vi "Remote Communication.vi"(4 "String":string, 5 "Max Mass":dbl, 6 "Error In":errorcluster, 7 "DC Param":u16, 8 "RT Parameter":T1 {"Expt"."Mass Range"."Resolution Type" items=["High/High", "Medium/Medium", "Low/Low", "High/Medium", "High/Low", "Medium/High", "Medium/Low", "Low/High", "Low/Medium"]}, 9 "Command":T7=enum."Start") -> (0 "Error Out":errorcluster, 1 "Data Array":i32[](array[numeric]), 2 "Info":string, 3 "Comm Error":bool)   [LabVIEW 2018]
doc: "This VI use TCP IP to communicate with RT"
uses:
  Type Defs/RT Command.ctl
  RT Parameters/RT Parameter.ctl
  RT Parameters/RT Experiments.ctl
  RT Parameters/RT Mass Range.ctl
  RT Parameters/RT Active Ch.ctl
  RT Parameters/RT Res Type.ctl
  RT Parameters/RT Run Mode.ctl
  Type Defs/Global Action.ctl
  Type Defs/TCP Packet Info.ctl
  Type Defs/RT Data.ctl
  FGVs/Global Variables.vi
panel:
  out "Number Matched":bool
  in  "IP Address":string
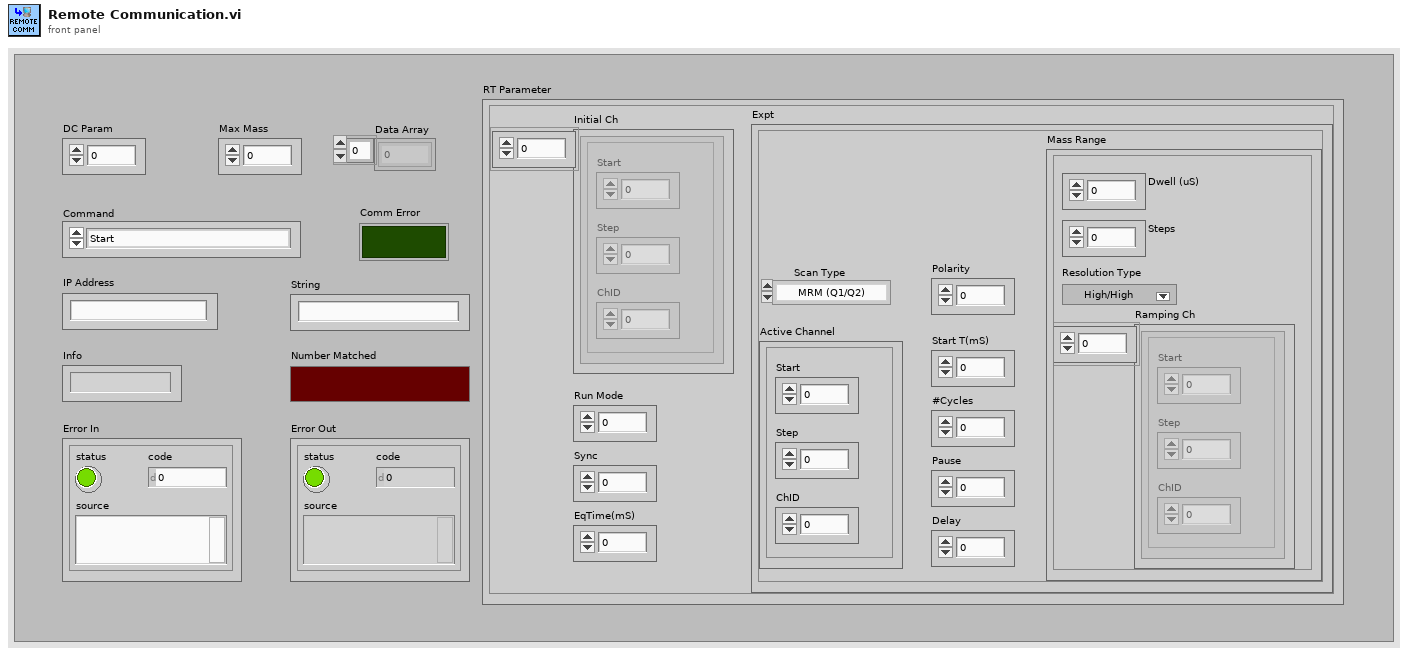
[diagram p1: front panel]
types:
  T1 = typedef "RT Parameter.ctl" = cluster{"Expt":T2, "Initial Ch":T4[], "Run Mode":i32, "Sync":u8, "EqTime(mS)":i32}
  T2 = typedef "RT Experiments.ctl" = cluster{"Mass Range":T3, "Active Channel":T4, "Scan Type":T6, "Polarity":u8, "Start T(mS)":i32, "#Cycles":i32, "Pause":i32, "Delay":i32}
  T3 = typedef "RT Mass Range.ctl" = cluster{"Ramping Ch":T4[], "Resolution Type":T5, "Steps":dbl, "Dwell (uS)":dbl}
  T4 = typedef "RT Active Ch.ctl" = cluster{"Start":dbl, "Step":dbl, "ChID":dbl}
  T5 = typedef "RT Res Type.ctl" = u16
  T6 = typedef "RT Run Mode.ctl" = enum16{"MRM (Q1/Q2)", "Q1 Scan", "Q1 SRM", "Q2 Scan", "Q2 SRM", "Product Scan", "Precursor Scan", "Neutral Loss", "Neutral Gain"}
  T7 = typedef "RT Command.ctl" = enum16{"xml Start Run", "xml Start Actual Run", "xml Stop Run", "xml Runtime Update", "xml Get Status", "xml Get Table", "xml Set Table", "xml Get Configuration", "xml System Status", "xml Set LC Input Logic", "xml Get Data", "xml Get Info", "Start", "StartActualRun", "Stop", "Runtime Update", "Get Data", "Get Info", "Get Status", "Get Param", "Get Config", "Get Table", "Read ADC", "Set Oscillator", "Update Config", "Update Table", "Set All Pol", "Set Pol and DC", "Set Max Mass", "Toggle RP", "Toggle EL", "Set PIC", "Initialize Turbo", "Send Turbo Comm", "Close Turbo", "P1", "P2", "P3", "Send Serial", "Set LC Out", "Get LC In", "Read VAC", "Test Table", "Toggle Power", "Get Startup", "Set Startup", "Get ADC Table", "Set ADC Table", "Get Brief Status", "Get Detail Status", "Auxiliary Update", "Set CC Logics", "Set CC Input Logics", "Ignore Error", "invalid"}
  T8 = typedef "TCP Packet Info.ctl" = cluster{"Packet Signature":string, "Sequence Number":i32, "Command":T7, "Data Message Size":u32, "Data Message Size":string, "Data Message":string, "Error Message Size":u32, "Error Message Size":string, "Error Message":string, "Checksum":u32, "Error Message":errorcluster, "Command ID":string}
  T9 = typedef "Global Action.ctl" = enum16{"Write", "Read"}
  T10 = typedef "RT Data.ctl" = cluster{"Info":string, "Data Array":i32[], "error out":errorcluster}
  T11 = typedef "Global Configrations.ctl" = cluster{"Model Name":enum16{"QSight 110", "QSight 120", "QSight 210", "QSight 220", "QSight 410", "QSight 420", "IONICS 3Q 110", "IONICS 3Q 120", "IONICS 3Q 210", "IONICS 3Q 220", "IONICS 3Q 310", "IONICS 3Q 320", "Simulation (Single Source)", "Simulation (Dual Source)"}, "RunType":u16, "Acquisition State":enum16{"Ready", "Busy", "Waiting"}, "InstrState":enum16{"Initializing", "Mass Spectrometer is Off", "Starting Up", "Turning Power Off", "Going to Standby", "Roughing Pump Ready", "Turning Turbo Off", "Turbo Startup", "Turbopump Ready", "Checking Vacuum", "Going to Ready", "Ready", "Running", "Source Standby", "Lost Communication", "Shutting Down", "Fault", "24V Standby", "Go to 24V Standby", "Turbopump Ready-Waiting"}, "Run Mode":enum16{"MRM (Q1/Q2)", "Q1 Scan", "Q1 SRM", "Q2 Scan", "Q2 SRM", "Product Scan", "Precursor Scan", "Neutral Loss", "Neutral Gain"}, "Configration":T12, "TCP ID":refnum<k5>, "DT":bool, "Dead Time (nS)":i32, "Single Source":bool, "ADC Tables":T14[]}
  T12 = typedef "Configration.ctl" = cluster{"Table":T13[], "Instrument":string[]}
  T13 = typedef "_RT Configuration 2.ctl" = cluster{"Name":string, "Ch#":u8, "Min":dbl, "Max":dbl, "Def+":dbl, "Def-":dbl, "Offset":dbl, "Slope":dbl, "Type":u8, "Description":string, "SettleT":dbl}
  T14 = typedef "ADC Table.ctl" = cluster{"Name":string, "Ch#":u8, "Min":dbl, "Max":dbl, "Def+":dbl, "Def-":dbl, "Offset":dbl, "Slope":dbl, "Type":u8, "Description":string, "SettleT":dbl}
  T15 = typedef "Global Parameters.ctl" = cluster{"Calibrations":cluster{"Q1 +ve":dbl[][], "Q2 +ve":dbl[][], "Q1 -ve":dbl[][], "Q2 -ve":dbl[][]}, "Resolution Q1":cluster{"High +ve":dbl[][], "Med +ve":dbl[][], "Low +ve":dbl[][], "High -ve":dbl[][], "Med -ve":dbl[][], "Low -ve":dbl[][]}, "Resolution Q2":cluster{"High +ve":dbl[][], "Med +ve":dbl[][], "Loe +ve":dbl[][], "High -ve":dbl[][], "Med -ve":dbl[][], "Low -ve":dbl[][]}, "MR Parameters":T16, "Mass":dbl[][], "Dwell":dbl[][], "Steps":i32[][], "Method Refnum":refnum<vi>}
  T16 = typedef "MR Parameters.ctl" = cluster{"Name":string, "Ch#":u8, "StartV":dbl, "StopV":dbl, "StepV":dbl, "Index":u8}
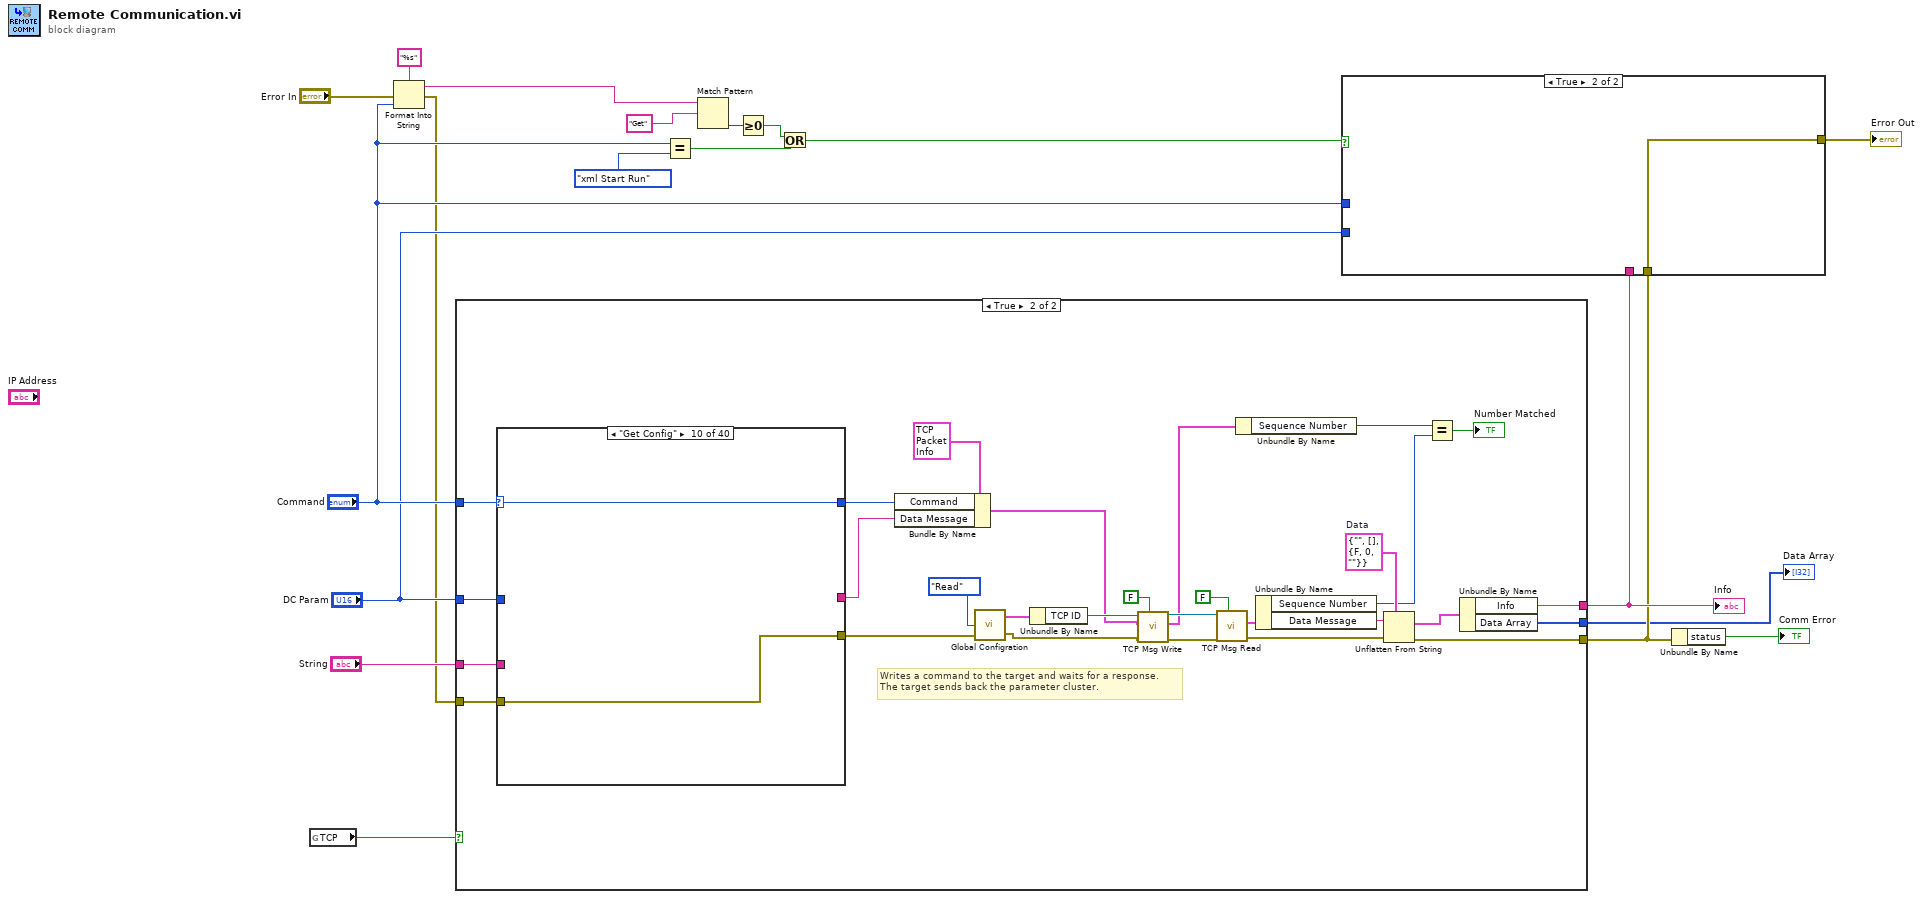
[diagram p0: block diagram]
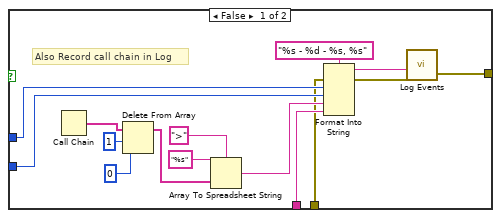
[diagram p2: hidden frame]
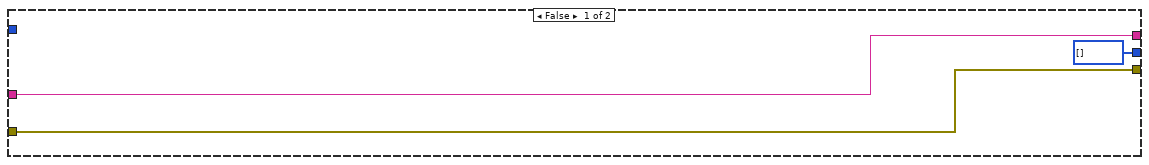
[diagram p3: hidden frame]
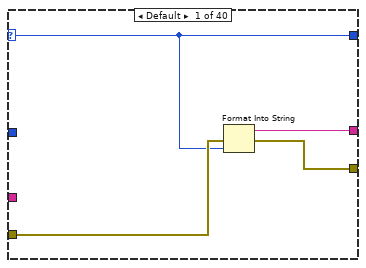
[diagram p4: hidden frame]
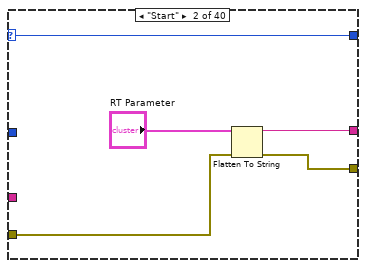
[diagram p5: hidden frame]
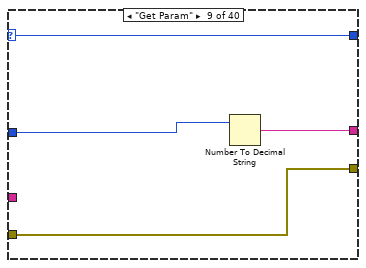
[diagram p12: hidden frame]
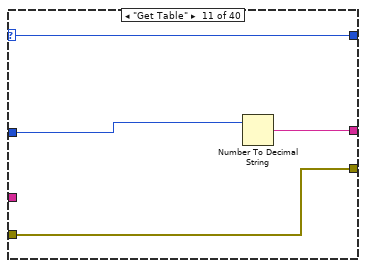
[diagram p13: hidden frame]
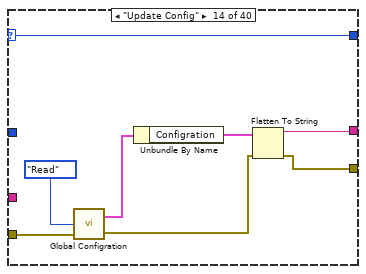
[diagram p16: hidden frame]
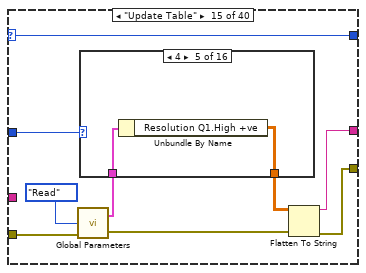
[diagram p17: hidden frame]
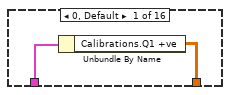
[diagram p18: hidden frame]
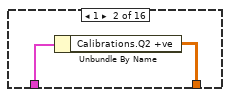
[diagram p19: hidden frame]
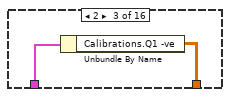
[diagram p20: hidden frame]
diagram:
  n1 = global read "Global Variables.vi" "TCP"() -> (w18:bool)
  n2 = Format Into String(format string="%s", error in="Error In", "Command") -> (resulting string=w6:string, error out=w5:errorcluster)  [unwired: 1 in]
  n3 = case shown="True" w18 {
    tunnel: "Command" -> [_ w51]
    tunnel: w5 -> [w22 w34]
    tunnel: "String" -> [w21 w48]
    tunnel: "DC Param" -> [_ w49]
    tunnel: [w22 w27] -> w3
    tunnel: [i32[] [] ("Data Array") w40] -> w1
    tunnel: [w21 w39] -> w8
    frame False {
    }
    frame True {
      w43 = T10 {"Info"="", "Data Array"=[], "error out"={"status"=FALSE, "code"=0, "source"=""}}  # Data
      # "Writes a command to the target and waits for a response.\nThe target sends back the parameter cluster."
      n4 = case shown="\"Get Config\"" w51 {
        selector: w51 -> [w53 w57 w62 w64 w65 w69 w71 w73 w77 w79 w80 w85 w88 w90 w98 w138 w143 w146 w153 w157 w160 w161 w165 w169 w174 w178 w180 w182 w183 w186 w191 w194 w196 w197 w200 w204 w205 w211 w215 w217]
        tunnel: [w53 w57 w62 w64 w65 w69 w71 w73 w77 w79 w80 w85 w88 w90 w98 w138 w143 w146 w153 w157 w160 w161 w165 w169 w174 w178 w180 w182 w183 w186 w191 w194 w196 w197 w200 w204 w205 w211 w215 w217] -> w50
        tunnel: w49 -> [_ _ _ _ _ _ _ _ w75 _ w82 _ _ _ w105 w140 w145 _ w150 w154 _ w163 w167 w171 _ w176 _ _ _ w188 _ _ _ _ _ _ _ w209 w213 w218]
        tunnel: w48 -> [_ _ _ _ w67 _ _ _ _ _ _ _ w87 _ _ _ _ _ _ _ w158 _ _ _ _ _ _ _ w185 _ _ w193 _ w199 w202 _ w206 _ _ _]
        tunnel: [w55 w60 _ _ w67 _ _ _ w76 _ w83 _ w87 w92 w100 w141 w144 w149 w151 w155 w158 w164 w168 w172 _ w177 _ _ w185 w189 _ w193 _ w199 w202 _ w206 w210 w214 w219] -> w47
        tunnel: w34 -> [w54 w58 w61 w63 w66 w68 w70 w72 w74 w78 w81 w84 w86 w93 w103 w139 w142 w147 w152 w156 w159 w162 w166 w170 w173 w175 w179 w181 w184 w187 w190 w192 w195 w198 w201 w203 w207 w208 w212 w216]
        tunnel: [w52 w59 w61 w63 w66 w68 w70 w72 w74 w78 w81 w84 w86 w91 w101 w139 w142 w147 w152 w156 w159 w162 w166 w170 w173 w175 w179 w181 w184 w187 w190 w192 w195 w198 w201 w203 w207 w208 w212 w216] -> w33
        frame Default {
          n5 = Format Into String(error in=w54, w53) -> (resulting string=w55:string, error out=w52:errorcluster)  [unwired: 2 in]
        }
        frame "Start" {
          n6 = Flatten To String(anything="RT Parameter", error in (no error)=w58) -> (data string=w60:string, error out=w59:errorcluster)  [unwired: 3 out]
        }
        frame "StartActualRun" {
        }
        frame "Stop" {
        }
        frame "Runtime Update" {
        }
        frame "Get Data" {
        }
        frame "Get Info" {
        }
        frame "Get Status" {
        }
        frame "Get Param" {
          n7 = Number To Decimal String(number=w75) -> (decimal integer string=w76:string)  [unwired: 1 out]
        }
        frame "Get Config" {
        }
        frame "Get Table" {
          n8 = Number To Decimal String(number=w82) -> (decimal integer string=w83:string)  [unwired: 1 out]
        }
        frame "Read ADC" {
        }
        frame "Set Oscillator" {
        }
        frame "Update Config" {
          n9 = call "Global Configration.vi"("Error In"=w93, "Action"=Global_Action."Read") -> ("Error Out"=w95:errorcluster, "Parameters Out"=w96:T11)  [unwired: 1 in]
          n10 = Unbundle By Name(w96) -> ("Configration"=w94:T12)
          n11 = Flatten To String(anything=w94, error in (no error)=w95) -> (data string=w92:string, error out=w91:errorcluster)  [unwired: 3 out]
        }
        frame "Update Table" {
          n12 = call "Global Parameters.vi"("Error In"=w103, "Action"=Global_Action."Read") -> ("Error Out"=w102:errorcluster, "Parameters Out"=w104:T15)  [unwired: 1 in]
          n13 = case shown="4" w105 {
            tunnel: w104 -> [w107 w109 w111 w112 w114 w116 w118 w120 w122 w124 w126 w128 w130 w132 w134 w136]
            tunnel: [w106 w108 w110 w113 w115 w117 w119 w121 w123 w125 w127 w129 w131 w133 w135 w137] -> w99
            frame 0, Default {
              n14 = Unbundle By Name(w107) -> ("Calibrations.Q1 +ve"=w106:dbl[][])
            }
            frame 1 {
              n15 = Unbundle By Name(w109) -> ("Calibrations.Q2 +ve"=w108:dbl[][])
            }
            frame 2 {
              n16 = Unbundle By Name(w111) -> ("Calibrations.Q1 -ve"=w110:dbl[][])
            }
            frame 3 {
              n17 = Unbundle By Name(w112) -> ("Calibrations.Q2 -ve"=w113:dbl[][])
            }
            frame 4 {
              n18 = Unbundle By Name(w114) -> ("Resolution Q1.High +ve"=w115:dbl[][])
            }
            frame 5 {
              n19 = Unbundle By Name(w116) -> ("Calibrations.Q1 +ve"=w117:dbl[][])
            }
            frame 6 {
              n20 = Unbundle By Name(w118) -> ("Calibrations.Q1 +ve"=w119:dbl[][])
            }
            frame 7 {
              n21 = Unbundle By Name(w120) -> ("Calibrations.Q1 +ve"=w121:dbl[][])
            }
            frame 8 {
              n22 = Unbundle By Name(w122) -> ("Calibrations.Q1 +ve"=w123:dbl[][])
            }
            frame 9 {
              n23 = Unbundle By Name(w124) -> ("Calibrations.Q1 +ve"=w125:dbl[][])
            }
            frame 10 {
              n24 = Unbundle By Name(w126) -> ("Calibrations.Q1 +ve"=w127:dbl[][])
            }
            frame 11 {
              n25 = Unbundle By Name(w128) -> ("Calibrations.Q1 +ve"=w129:dbl[][])
            }
            frame 12 {
              n26 = Unbundle By Name(w130) -> ("Calibrations.Q1 +ve"=w131:dbl[][])
            }
            frame 13 {
              n27 = Unbundle By Name(w132) -> ("Calibrations.Q1 +ve"=w133:dbl[][])
            }
            frame 14 {
              n28 = Unbundle By Name(w134) -> ("Calibrations.Q1 +ve"=w135:dbl[][])
            }
            frame 15 {
              n29 = Unbundle By Name(w136) -> ("Calibrations.Q1 +ve"=w137:dbl[][])
            }
          }
          n30 = Flatten To String(anything=w99, error in (no error)=w102) -> (data string=w100:string, error out=w101:errorcluster)  [unwired: 3 out]
        }
        frame "Set All Pol" {
          n31 = Type Cast(x=w140) -> (*(type *) &x=w141:string)  [unwired: 1 in]
        }
        frame "Set Pol and DC" {
          n32 = Type Cast(x=w145) -> (*(type *) &x=w144:string)  [unwired: 1 out]
        }
        frame "Set Max Mass" {
          n33 = Type Cast(x="Max Mass") -> (*(type *) &x=w149:string)  [unwired: 1 in]
        }
        frame "Toggle RP" {
          n34 = Number To Decimal String(number=w150) -> (decimal integer string=w151:string)  [unwired: 1 out]
        }
        frame "Toggle EL" {
          n35 = Number To Decimal String(number=w154) -> (decimal integer string=w155:string)  [unwired: 1 out]
        }
        frame "Set PIC" {
        }
        frame "P1" {
          n36 = Type Cast(x=w163) -> (*(type *) &x=w164:string)  [unwired: 1 in]
        }
        frame "P2" {
          n37 = Type Cast(x=w167) -> (*(type *) &x=w168:string)  [unwired: 1 in]
        }
        frame "P3" {
          n38 = Type Cast(x=w171) -> (*(type *) &x=w172:string)  [unwired: 1 in]
        }
        frame "Send Serial" {
        }
        frame "Set LC Out" {
          n39 = Type Cast(x=w176) -> (*(type *) &x=w177:string)  [unwired: 1 in]
        }
        frame "Get LC In" {
        }
        frame "Read VAC" {
        }
        frame "Test Table" {
        }
        frame "Toggle Power" {
          n40 = Number To Decimal String(number=w188) -> (decimal integer string=w189:string)  [unwired: 1 out]
        }
        frame "Get Startup" {
        }
        frame "Set Startup" {
        }
        frame "Get ADC Table" {
        }
        frame "Set ADC Table" {
        }
        frame "Get Brief Status" {
        }
        frame "Get Detail Status" {
        }
        frame "Auxiliary Update" {
        }
        frame "Set CC Logics" {
          n41 = Type Cast(x=w209) -> (*(type *) &x=w210:string)  [unwired: 1 in]
        }
        frame "Set CC Input Logics" {
          n42 = Type Cast(x=w213) -> (*(type *) &x=w214:string)  [unwired: 1 in]
        }
        frame "Ignore Error" {
          n43 = Number To Decimal String(number=w218) -> (decimal integer string=w219:string)  [unwired: 1 out]
        }
      }
      n44 = Bundle By Name(cluster=T8 {"Packet Signature"="", "Sequence Number"=0, "Command"=enum."Get Info", "Data Message Size"=0, "Data Message Size"="", "Data Message"="", "Error Message Size"=0, "Error Message Size"="", "Error Message"="", "Checksum"=0, "Error Message"={"status"=FALSE, "code"=0, "source"=""}, "Command ID"=""} ("Packet Info In Out 2"), "Command"=w50, "Data Message"=w47) -> (w36:T8)
      n45 = call "Global Configration.vi"("Error In"=w33, "Action"=Global_Action."Read") -> ("Error Out"=w38:errorcluster, "Parameters Out"=w46:T11)  [unwired: 1 in]
      n46 = Unbundle By Name(w46) -> ("TCP ID"=w37:refnum<k5>)
      n47 = call "TCP Msg Write.vi"("RT"=FALSE, "error in"=w38, "Packet Info In"=w36, "connection ID In"=w37) -> ("error out"=w32:errorcluster, "Packet Info In Out"=w24:T8, "connection ID out"=w28:refnum<k5>)  [unwired: 5 in]
      n48 = call "TCP Msg Read.vi"("RT"=FALSE, "error in"=w32, "connection ID"=w28) -> ("error out"=w30:errorcluster, "Packet Info"=w31:T8)  [unwired: 5 in, 2 out]
      n49 = Unbundle By Name(w24) -> ("Sequence Number"=w25:i32)
      n50 = Unbundle By Name(w31) -> ("Sequence Number"=w23:i32, "Data Message"=w42:string)
      n51 = Unflatten From String(type=w43, binary string=w42, error in (no error)=w30) -> (value=w41:T10, error out=w27:errorcluster)  [unwired: 3 out]
      n52 = Equal?(x=w25, y=w23) -> (x = y?=→"Number Matched":bool)
      n53 = Unbundle By Name(w41) -> ("Info"=w39:string, "Data Array"=w40:i32[])
    }
  }
  "Info" <- w8
  "Data Array" <- w1
  n54 = Equal?(x="Command", y=RT_Command."xml Start Run" ("RT Command")) -> (x = y?=w13:bool)
  n55 = Match Pattern(string=w6, regular expression="Get") -> (offset past match=w15:i32)  [unwired: 4 out]
  n56 = Greater Or Equal To 0?(x=w15) -> (x >= 0?=w14:bool)
  n57 = Or(x=w14, y=w13) -> (x .or. y?=w11:bool)
  n58 = case shown="True" w11 {
    tunnel: "Command" -> [w226 _]
    tunnel: "DC Param" -> [w225 _]
    tunnel: w8 -> [w224 _]
    tunnel: w3 -> [w222 w235]
    tunnel: [w220 w235] -> w7
    frame False {
      # "Also Record call chain in Log"
      n59 = Call Chain() -> (call chain=w231:string[])
      n60 = Delete From Array(array=w231, length=1, index=0) -> (array with subset deleted=w228:string[])  [unwired: 1 out]
      n61 = Array To Spreadsheet String(delimiter (Tab)=">", array=w228, 3:"%s" ("format string")) -> (spreadsheet string=w227:string)
      n62 = Format Into String(format string="%s - %d - %s, %s", error in=w222, w226, w225, w227, w224) -> (resulting string=w223:string, error out=w221:errorcluster)  [unwired: 1 in]
      n63 = call "Log Events.vi"("Error In"=w221, "Event"=w223) -> ("Error Out"=w220:errorcluster)  [unwired: 4 in, 1 out]
    }
    frame True {
    }
  }
  "Error Out" <- w7
  n64 = Unbundle By Name(w3) -> ("status"=→"Comm Error":bool)
